vi "GetProviderName.vi"(0 "ClassWriterGOOP300 in":refnum<class "ClassWriterGOOP300.lvclass">, 5 "error in (no error)":errorcluster) -> (14 "ClassWriterGOOP300 out":refnum<class "ClassWriterGOOP300.lvclass">, 15 "ProviderName":string, 17 "TranslatedProviderName":string, 19 "error out":errorcluster)   [LabVIEW 2020, in "ClassWriterGOOP300.lvclass"]
uses:
  <resource>/Framework/Providers/Open_GDS/ClassProviders/Provider_EndevoGOOP300/ClassWriterGOOP300_class/ClassWriterGOOP300.lvclass
  <resource>/Framework/Providers/Open_GDS/ClassProviders/Provider_EndevoGOOP300/EndevoProviderName.ctl
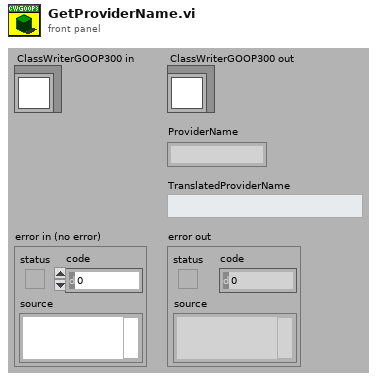
[diagram p1: front panel]
types:
  T1 = typedef "EndevoProviderName.ctl" = enum16{"EndevoGOOP300"}
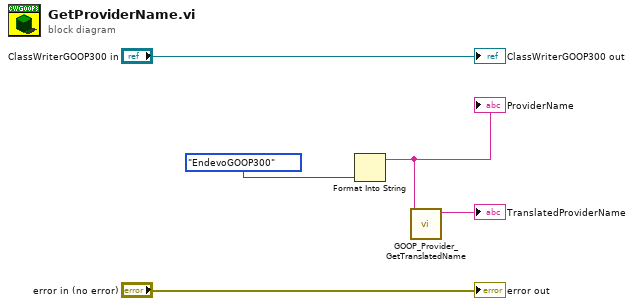
[diagram p0: block diagram]
diagram:
  n1 = Format Into String(EndevoProviderName."EndevoGOOP300" ("ProviderName")) -> (resulting string=w1:string)  [unwired: 3 in, 1 out]
  "ProviderName" <- w1
  n2 = call <resource>:"GOOP_Provider_GetTranslatedName.vi"("ProviderName"=w1) -> ("TranslatedName"=→"TranslatedProviderName":string)  [unwired: 10 in]
  "ClassWriterGOOP300 out" <- "ClassWriterGOOP300 in"
  "error out" <- "error in (no error)"
